vi "FTW-CodeGen-Callback-FindGObjects.vi"(4 "context in":variant, 5 "objref":refnum<vi>) -> (1 "context out":variant, 2 "traverse flags":i32 format="0x%08x")   [LabVIEW 2015]
panel:
  # "Inputs"
  # "Outputs"
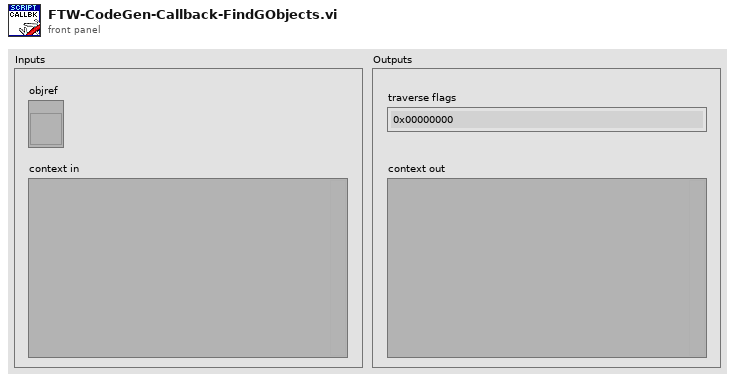
[diagram p1: front panel]
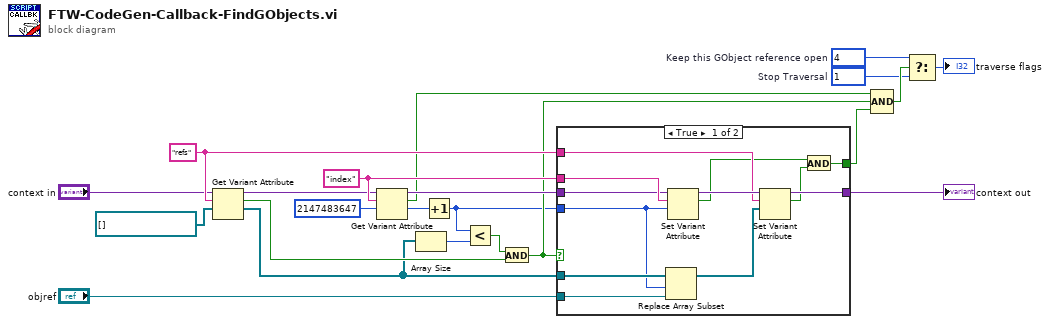
[diagram p0: block diagram]
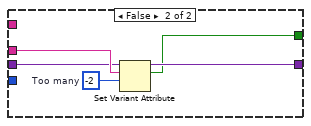
[diagram p2: hidden frame]
diagram:
  w21 = "refs" ("name")
  w22 = "index" ("name")
  w10 = 4  # Keep this GObject reference open
  w11 = 1  # Stop Traversal
  n1 = Get Variant Attribute(Variant="context in", name=w21, default value (empty Variant)=refnum<vi>[] [] ("initialized array")) -> (duplicate Variant=w19:variant, found=w6:bool, value=w1:refnum<vi>[])  [unwired: 1 in, 1 out]
  n2 = Get Variant Attribute(Variant=w19, name=w22, default value (empty Variant)=2147483647) -> (duplicate Variant=w18:variant, found=w13:bool, value=w4:i32)  [unwired: 1 in, 1 out]
  n3 = Array Size(array=w1) -> (size(s)=w14:i32)
  n4 = Increment(x=w4) -> (x+1=w3:i32)
  n5 = Less?(x=w3, y=w14) -> (x < y?=w7:bool)
  n6 = And(x=w7, y=w6) -> (x .and. y?=w5:bool)
  n7 = case shown="True" w5 {
    tunnel: w22 -> [w34 w39]
    tunnel: w21 -> [w32 _]
    tunnel: w18 -> [w31 w38]
    tunnel: [w30 w37] -> w17
    tunnel: w3 -> [w24 _]
    tunnel: [w27 w35] -> w8
    tunnel: w1 -> [w26 _]
    tunnel: "objref" -> [w23 _]
    frame True {
      n8 = Replace Array Subset(array=w26, new element=w23, index=w24) -> (w25:refnum<vi>[])
      n9 = Set Variant Attribute(Variant=w31, name=w34, value=w24) -> (Variant out=w33:variant, replaced=w28:bool)  [unwired: 1 in, 1 out]
      n10 = Set Variant Attribute(Variant=w33, name=w32, value=w25) -> (Variant out=w30:variant, replaced=w29:bool)  [unwired: 1 in, 1 out]
      n11 = And(x=w28, y=w29) -> (x .and. y?=w27:bool)
    }
    frame False {
      w36 = -2  # Too many
      n12 = Set Variant Attribute(Variant=w38, name=w39, value=w36) -> (Variant out=w37:variant, replaced=w35:bool)  [unwired: 1 in, 1 out]
    }
  }
  "context out" <- w17
  n13 = Compound Arithmetic op=AND(w13, w5, w8) -> (w12:bool)
  n14 = Select(t=w10, s=w12, f=w11) -> (s? t:f=→"traverse flags":i32)
